vi "Multiplier 3.vi"   [LabVIEW 2009]
doc: "Little contemplated fact: This vi is actually a simple processor."
uses:
  <vilib>/Platform/TimedLoop/XDataNode/XDataNode.xnode
  <vilib>/Platform/TimedLoop/XDataNode/loadlvalarms.vi
  <vilib>/Platform/TimedLoop/XDataNode/timing_clust.ctl
  <vilib>/Platform/TimedLoop/XDataNode/nitl_modes.ctl
  <vilib>/Platform/TimedLoop/XDataNode/wakeup.ctl
  Motor Control Global.vi
  <vilib>/rvi/DataTransferAndStorage/Container/XNode/niFpgaContainer.xnode
  <vilib>/rvi/DataTransferAndStorage/Container/Common/niFpgaContainerMethod.ctl
  <vilib>/rvi/DataTransferAndStorage/Container/Common/niFpgaContainerExecOnDevCompGetState.vi
  <vilib>/rvi/DataTransferAndStorage/Container/Common/niFpgaContainerMetaDataKey.ctl
  <vilib>/rvi/FIFO/Fifo_Resource/nirvififoUniquifyingName.vi
  <vilib>/rvi/interface/RandomDataEmulation/niFpgaRandomDataHandleErrors.vi
  <vilib>/rvi/interface/RandomDataEmulation/nirviRandomDataFPGAFIFO.vi
  <vilib>/rvi/DataTransferAndStorage/Container/Common/niFpgaTransferTypeControl.ctl
  <vilib>/rvi/DataTransferAndStorage/FIFO/niFpgaPeerToPeerStreamState.ctl
  <vilib>/rvi/eio/common/nirviEmuReportErrorAndStop.vi
  <vilib>/rvi/FXPMathLib/FxpMul/XNode/nifxpmath_Multiplier.xnode
  <vilib>/rvi/FXPMathLib/FxpMul/subVIs/nifxpmath_Mul_SimConfig.ctl
  <vilib>/fxp/LVFixedPointQuantizationPolicyTypeDef.ctl
  <vilib>/fxp/LVFixedPointOverflowPolicyTypeDef.ctl
  <vilib>/rvi/FXPMathLib/FxpMul/simVIs/DllFxpMulTemp_sub.vi
  <vilib>/rvi/Memory/Memory_Emulation/nirvimemoryEmulationManagerCache_GetValue.vi
  <vilib>/rvi/Memory/Memory_Emulation/nirvimemoryEmulationManagerCache_InsertValue.vi
  <vilib>/Utility/error.llb/Clear Errors.vi
  <vilib>/rvi/Memory/Memory_Emulation/nirvimemoryEmulationManagerCache_SetValue.vi
  <vilib>/Platform/TimedLoop/XDataNode/XDNodeRunTimeDep.lvlib
types:
  T1 = typedef "niFpgaContainerMetaDataKey.ctl" = enum16{"FPGA FIFO", "FPGA Memory", "FPGA Register"}
  T2 = typedef "niFpgaContainerMethod.ctl" = enum16{"Write", "Read", "Clear", "Get Number of Elements to Write", "Get Number of Elements to Read", "Enable", "Disable", "Flush and Disable", "Get Stream State"}
  T3 = typedef "niFpgaTransferTypeControl.ctl" = enum16{"Target-Scoped", "Host to Target - DMA", "Target to Host - DMA", "Peer to Peer Reader", "Peer to Peer Writer", "Bidirectional"}
  T4 = typedef "niFpgaPeerToPeerStreamState.ctl" = enum16{"Unlinked", "Disabled", "Enabled", "Flushing"}
  T5 = typedef "XDNodeRunTimeDep.lvlib/timing_clust.ctl" = cluster{"Expected End [f-1]":u64, "Actual End [f-1]":u64, "Finished Late? [f-1]":bool, "Expected End [i-1]":u64, "Actual End [i-1]":u64, "Finished Late? [i-1]":bool, "Expected Start [i]":u64, "Actual Start [i]":u64, "Expected Start [f]":u64, "Actual Start [f]":u64, "Source Name":string, "Structure Name":string, "Period":i64, "Deadline":i64, "Offset":i64, "Start":i64, "Priority":i32, "Timeout":i32, "Mode":T6, "Wakeup Reason":T7, "Error":errorcluster, "Source Type":string, "Secondary Source Type":string, "Global End Time":u64, "Global Start Time":u64, "Frame Duration":u64, "Iteration Duration":u64, "Assigned CPU":i32, "I/O Scan Engine Mode":u32}
  T6 = typedef "XDNodeRunTimeDep.lvlib/nitl_modes.ctl" = enum32{"No Change", "Process missed periods, maintain original phase", "Discard missed periods, maintain original phase", "Process missed periods, ignore original phase", "Discard missed periods, ignore original phase"}
  T7 = typedef "XDNodeRunTimeDep.lvlib/wakeup.ctl" = enum32{"Normal", "Aborted", "Asynchronous wakeup", "Timing source error", "Timed loop error", "Timeout"}
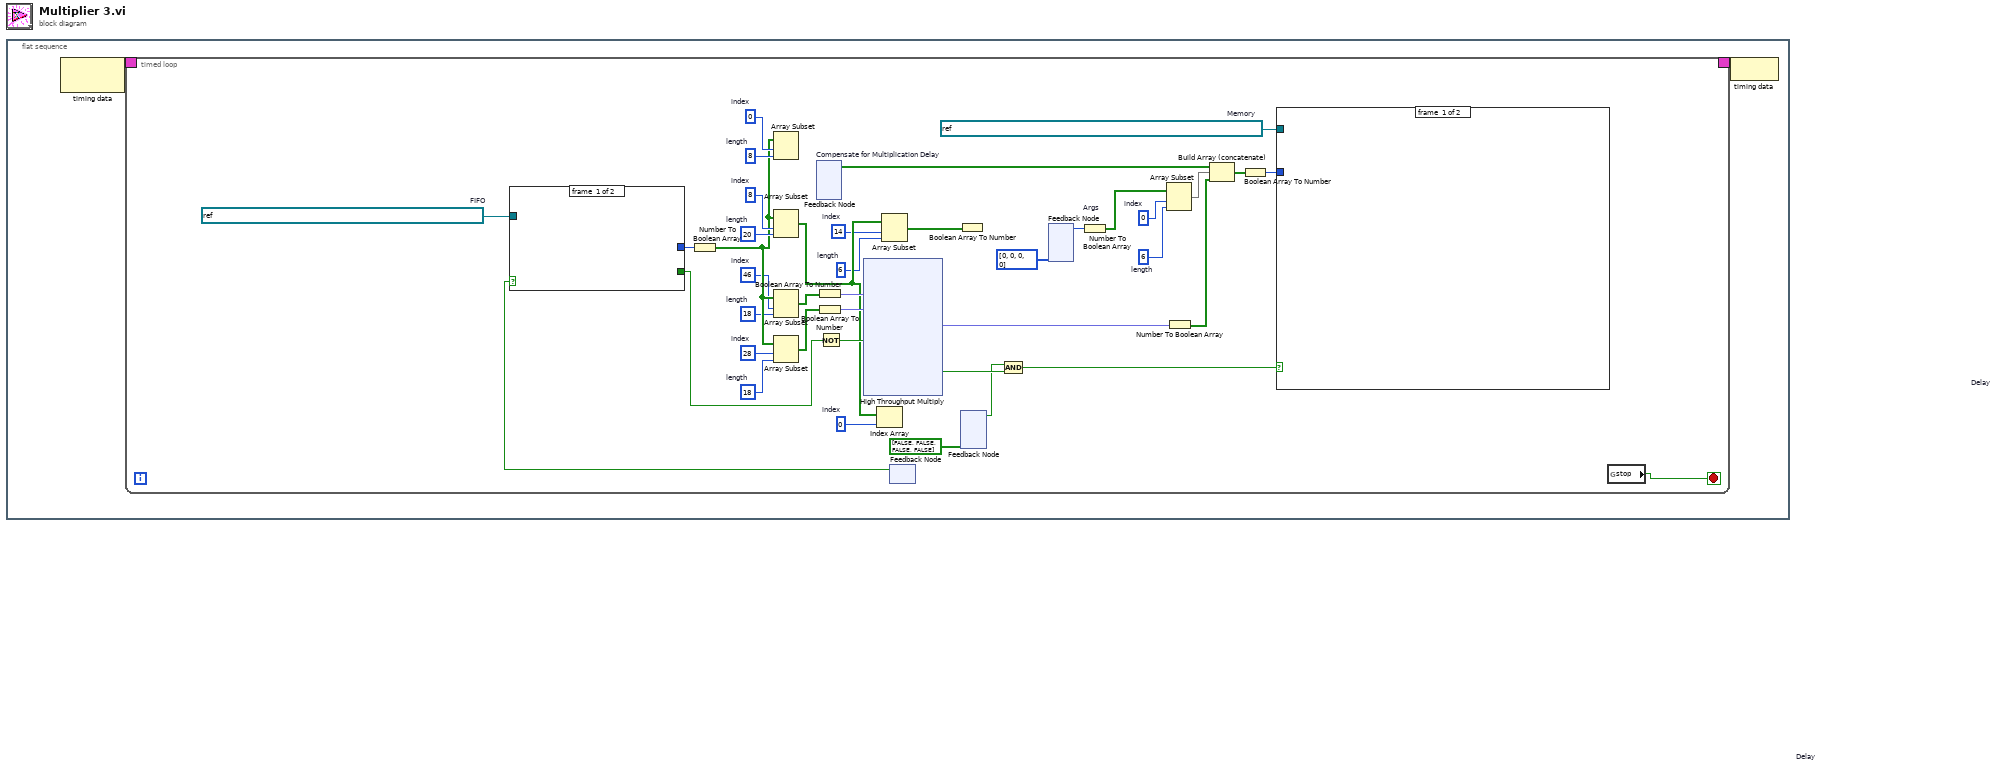
[diagram p0: block diagram]
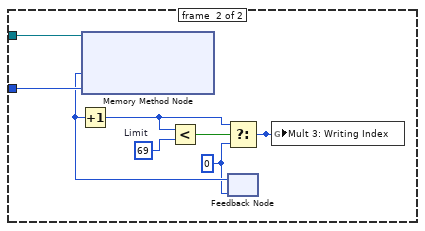
[diagram p2: hidden frame]
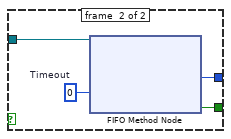
[diagram p3: hidden frame]
diagram:
  n1 = flat-sequence {
    frame #0 {
      n2 = node-c288() -> (w2:T5)  [unwired: 1 in]
      n3 = timed-loop {
        timing: w2 -> [_]
        timing-out: [_] -> w1
        stop <- w19 stop-if-true
        w4 = refnum<k21> "Multiplier 3 FIFO In : [8b Identifier; 20b args; 18b fxp; 18b fxp]"  # FIFO
        w3 = refnum<k21> "Multiplier 3 Block Memory Out: [8b Identifier; 6b args; 18b fxp output]"  # Memory
        w5 = 6  # length
        w6 = 0  # index
        w13 = 6  # length
        w14 = 14  # index
        w21 = 0  # index
        w35 = 18  # length
        w36 = 46  # index
        w38 = 18  # length
        w39 = 28  # index
        w40 = 20  # length
        w41 = 8  # index
        w42 = 8  # length
        w43 = 0  # index
        n4 = feedback #1 "Compensate for Multiplication Delay"() -> (w22:bool[])  [unwired: 1 in]
        n5 = feedback #2() -> (w26:bool)  [unwired: 1 in]
        n6 = case shown="True" w26 {
          tunnel: w4 -> [_ w254]
          tunnel: [_ w253] -> w46
          tunnel: [_ w252] -> w44
          frame #0 {
          }
          frame #1 {
            w251 = 0  # Timeout
            n7 = xnode ("FIFO Method Node")("Timeout"=w251, "FIFO In"=w254) -> ("Element"=w252:u64, "Timed Out?"=w253:bool)  [unwired: 1 out]
          }
        }
        n8 = Number To Boolean Array(number=w44) -> (Boolean array=w37:bool[])
        n9 = Array Subset(array=w37, index=w43, length=w42) -> (w30:bool[])
        n10 = Array Subset(array=w37, index=w41, length=w40) -> (w15:bool[])
        n11 = Array Subset(array=w37, index=w36, length=w35) -> (w34:bool[])
        n12 = Array Subset(array=w37, index=w39, length=w38) -> (w33:bool[])
        n13 = Boolean Array To Number(Boolean array=w34) -> (number=w24:fxp<+/-,18,1>)
        n14 = Boolean Array To Number(Boolean array=w33) -> (number=w23:fxp<+/-,18,1>)
        n15 = Not(x=w46) -> (.not. x?=w45:bool)
        n16 = xnode "High Throughput Multiply"("x"=w24, "y"=w23, "input valid"=w45) -> ("x*y"=w32:fxp<+/-,18,1>, "output valid"=w25:bool, "ready for input"=w27:bool)  [unwired: 1 in]
        n17 = Index Array(array=w15, index=w21) -> (element=w18:bool)
        n18 = Array Subset(array=w15, index=w14, length=w13) -> (w12:bool[])
        n19 = Boolean Array To Number(Boolean array=w12) -> (number=w11:u8)
        n20 = feedback #3 "Delay"(bool[] [FALSE, FALSE, FALSE, FALSE]) -> (w17:bool)
        n21 = And(x=w17, y=w25) -> (x .and. y?=w20:bool)
        n22 = feedback #4 "Delay"(u8[] [0, 0, 0, 0]) -> (w9:u8)
        n23 = Number To Boolean Array "Args"(number=w9) -> (Boolean array=w8:bool[])
        n24 = Array Subset(array=w8, index=w6, length=w5) -> (w7:bool[])
        n25 = Number To Boolean Array(number=w32) -> (Boolean array=w29:bool[])
        n26 = Build Array (concatenate)(w22, w7, w29) -> (w31:bool[])
        n27 = Boolean Array To Number(Boolean array=w31) -> (number=w28:u32)
        n28 = case shown="True" w20 {
          tunnel: w3 -> [_ w54]
          tunnel: w28 -> [_ w50]
          frame #0 {
          }
          frame #1 {
            w52 = u32 69  # Limit
            w47 = u32 0
            n29 = feedback #5(w47) -> (w49:u32)
            n30 = Increment(x=w49) -> (x+1=w53:u32)
            n31 = xnode ("Memory Method Node")("Address"=w49, "Data"=w50, "Memory In"=w54) -> ()  [unwired: 1 out]
            n32 = Less?(x=w53, y=w52) -> (x < y?=w51:bool)
            n33 = Select(t=w53, s=w51, f=w47) -> (s? t:f=w48:u32)
            n34 = global write "Motor Control Global.vi" "Mult 3: Writing Index"(w48) -> ()
          }
        }
        n35 = global read "Motor Control Global.vi" "stop"() -> (w19:bool)
      }
      n36 = node-c288(w1) -> ()
    }
  }
